vi "brc_daq_get_parameters.vi"(5 "error in (no error)":errorcluster, 6 "mHandle":i32) -> (14 "sample_rate":dbl, 15 "coupling_mode":i32, 16 "current":dbl, 19 "error out":errorcluster)   [LabVIEW 2019, in "BRC-DAQ x86.lvlib"]
uses:
  BRC-DAQ x86.lvlib
  DLL/brc_daq_sdk.dll
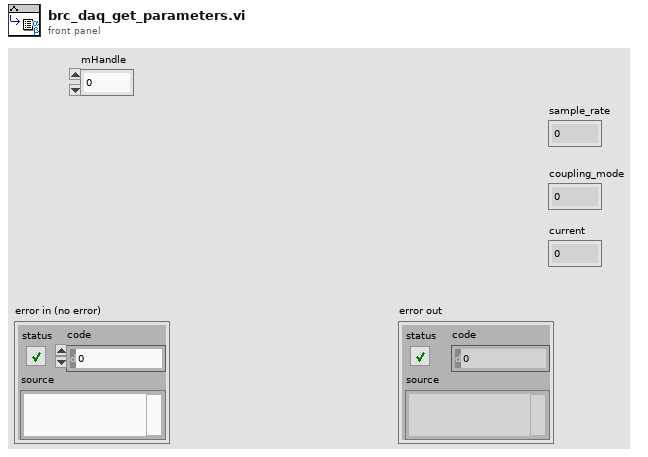
[diagram p1: front panel]
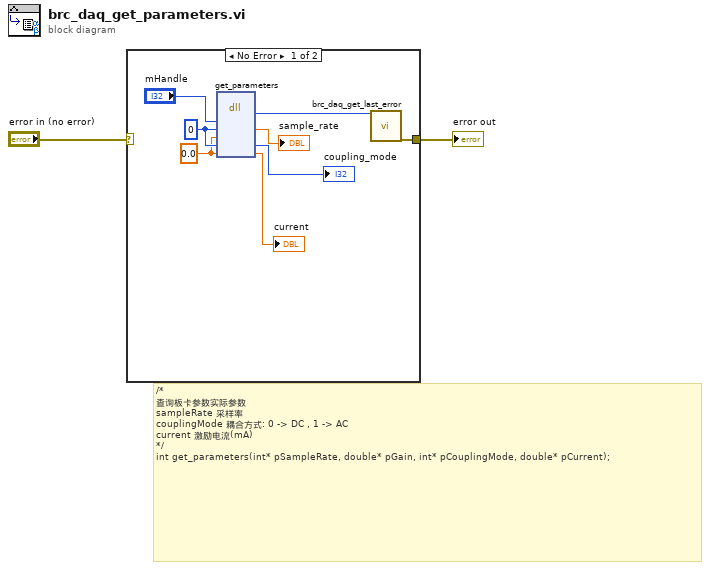
[diagram p0: block diagram]
diagram:
  # "/*\n查询板卡参数实际参数\nsampleRate 采样率\ncouplingMode 耦合方式: 0 -> DC , 1 -> AC\ncurrent 激励电流(mA)\n*/\nint get_parameters(int* pSampleRate, double* pGain, int* pCouplingMode, double* pCurrent);"
  n1 = case shown="No Error" "error in (no error)" {
    selector: "error in (no error)" -> [_ w11]
    tunnel: [w6 w11] -> w2
    frame No Error {
      w5 = 0 ("sampleRate")
      w4 = 0.0 ("pGain")
      n2 = dll-call lib="E:/01 BRC project/04BRC-daq/04 Drive/BRC-DAQ/DAQ-x64/DLL/brc_daq_sdk.dll" fn="get_parameters"("mHandle"="mHandle", "sampleRate"=w5, "Gain"=w4, "couplingMode"=w5, "current"=w4) -> ("return type"=w7:i32, "sampleRate"=→"sample_rate":dbl, "couplingMode"=→"coupling_mode":i32, "current"=→"current":dbl)  [unwired: 5 in, 2 out]
      n3 = call "brc_daq_get_last_error.vi"("return_value"=w7) -> ("error out"=w6:errorcluster)  [unwired: 18 in]
    }
    frame Error {
    }
  }
  "error out" <- w2
